vi "PH_TKTDS-30xx.set Channel GUI Element.vi"(0 "i ref in":refnum<vi>, 2 "GUI Element Name":string="N/A", 3 "Channel Config":T1={"Channel Name"="CH1", "Input Impedance"="MEG", "Max Input Frequency"="TWENTY", "Vertical Coupling"=1, "Channel Enabled"=TRUE, "Probe Attenuation"=1.0, "Vertical Range"=100.0, "Vertical Offset"=0.0, "Waveform Limits"={"Start"=1, "End"=10000}} {"Vertical Offset" format="%#_6p"; "Vertical Range" items=["1mV"=0.001, "2mV"=0.002, "5mV"=0.005, "10mV"=0.01, "20mV"=0.02, "50mV"=0.05, "100mV"=0.1, "200mV"=0.2, "500mV"=0.5, "1V"=1.0]; "Probe Attenuation" format="%#.2f"}, 5 "error in":errorcluster) -> (14 "i ref out":refnum<vi>, 19 "error out":errorcluster)   [LabVIEW 2014, in "PH_TKTDS-30xx.lvlib"]
doc: "If the reference is valid, the incoming data are set to the GUI."
uses:
  PH_TKTDS-30xx.lvlib
  PH_TKTDS-30xx.Channel Config.ctl
  PH_TKTDS-30xx.Waveform Limits.ctl
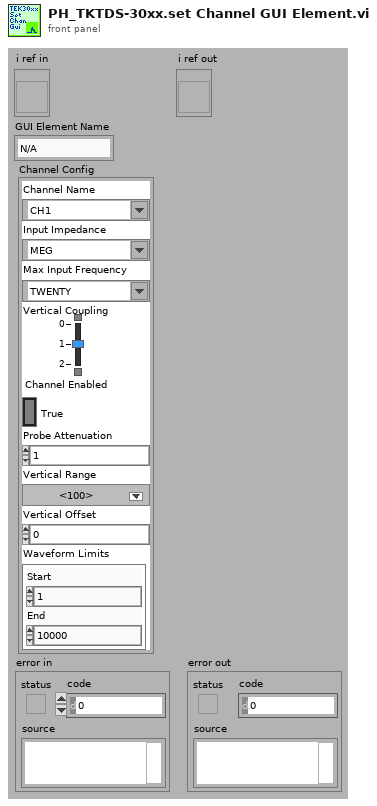
[diagram p1: front panel]
types:
  T1 = typedef "PH_TKTDS-30xx.lvlib/PH_TKTDS-30xx.Channel Config.ctl" = cluster{"Channel Name":string, "Input Impedance":string, "Max Input Frequency":string, "Vertical Coupling":i32, "Channel Enabled":bool, "Probe Attenuation":dbl, "Vertical Range":dbl, "Vertical Offset":dbl, "Waveform Limits":T2}
  T2 = typedef "PH_TKTDS-30xx.lvlib/PH_TKTDS-30xx.Waveform Limits.ctl" = cluster{"Start":i32, "End":i32}
  T3 = typedef "PH_TKTDS-30xx.lvlib/PH_TKTDS-30xx.i attribute.ctl" = cluster{"Default VISA Resource":string, "VISA Resource Name":refnum<visa-resource-name>, "Revision":cluster{"Instrument Driver":string, "Instrument Firmware":string}, "Selftest":cluster{"Result":u32, "Message":string}, "Channels":T1[], "Trigger Configuration":T4, "Acquisition Configuration":T5, "Fetched Waveforms":T6[], "GUI Refs":T7, "State":T8, "Error Message":string, "Allow Prdc Loop?":bool}
  T4 = typedef "PH_TKTDS-30xx.lvlib/PH_TKTDS-30xx.Trigger Config.ctl" = cluster{"Source":string, "Slope":i32, "Level [V]":dbl}
  T5 = typedef "PH_TKTDS-30xx.lvlib/PH_TKTDS-30xx.Acquisition Config.ctl" = cluster{"Time base":dbl, "Record Length":u16, "Start Time":dbl, "Type":i32, "Continuous":bool}
  T6 = typedef "PH_TKTDS-30xx.lvlib/PH_TKTDS-30xx.fetched Waveform.ctl" = cluster{"Source":string, "Actual Points":u32, "Initial X":dbl, "X Increment":dbl, "Waveform Array":dbl[]}
  T7 = typedef "PH_TKTDS-30xx.lvlib/PH_TKTDS-30xx.GUI Refs.ctl" = cluster{"Trigger":refnum<vi>, "Acquisition":refnum<vi>, "State":refnum<vi>, "Delete":refnum<vi>, "Channel to be positioned":refnum<vi>, "Postion":refnum<vi>, "Display Intensity":refnum<vi>, "VISA Resource":refnum<vi>, "Channels":refnum<vi>[], "Graphs":refnum<vi>[]}
  T8 = typedef "PH_StatusHandler.lvlib/PH_StatusHandler.Status.ctl" = i16
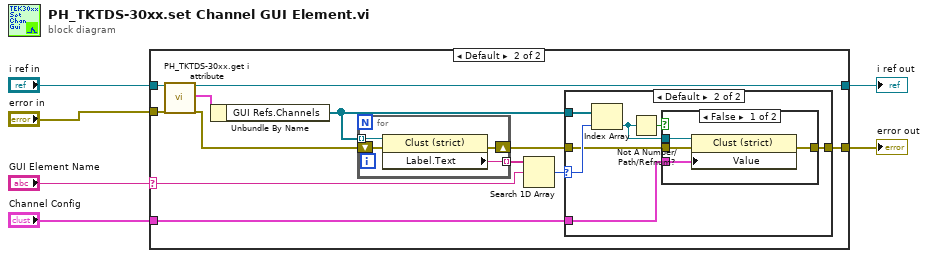
[diagram p0: block diagram]
diagram:
  n1 = case shown="Default" "GUI Element Name" {
    selector: "GUI Element Name" -> [_ w9]
    tunnel: "Channel Config" -> [_ w16]
    tunnel: [w7 w15] -> w5
    tunnel: "error in" -> [w7 w12]
    tunnel: "i ref in" -> [w8 w11]
    tunnel: [w8 w10] -> w2
    frame "", "N/A" {
    }
    frame Default {
      n2 = call "PH_TKTDS-30xx.get i attribute.vi"("i ref in"=w11, "error in (no error)"=w12) -> ("i ref out"=w10:refnum<vi>, "i attribute"=w14:T3, "error out"=w13:errorcluster)  [unwired: 15 in]
      n3 = Unbundle By Name(w14) -> ("GUI Refs.Channels"=w18:refnum<vi>[])
      n4 = for {
        tunnel: w18 -> [w37] mode=indexing
        tunnel: [w36] -> w20 mode=indexing
        shift-right: [w35] -> w17
        shift-left: w13 -> [w34]
        n5 = property class="Clust (strict)"(reference=w37, error in=w34) -> (error out=w35:errorcluster, "Label.Text"=w36:string)  [unwired: 1 out]
      }
      n6 = Search 1D Array(1D array=w20, element=w9) -> (index of element=w19:i32)  [unwired: 1 in]
      n7 = case shown="Default" w19 {
        selector: w19 -> [_ w27]
        tunnel: w18 -> [_ w28]
        tunnel: w17 -> [w21 w25]
        tunnel: w16 -> [_ w24]
        tunnel: [w21 w23] -> w15
        frame -1 {
        }
        frame Default {
          n8 = Index Array(array=w28, index=w27) -> (element=w26:refnum<vi>)
          n9 = Not A Number/Path/Refnum?(number/path/refnum=w26) -> (NaN/Path/Refnum?=w22:bool)
          n10 = case shown="False" w22 {
            tunnel: w25 -> [w32 w33]
            tunnel: [w31 w33] -> w23
            tunnel: w26 -> [w30 _]
            tunnel: w24 -> [w29 _]
            frame False {
              n11 = property class="Clust (strict)"(reference=w30, error in=w32, "Value"=w29) -> (error out=w31:errorcluster)  [unwired: 1 out]
            }
            frame True {
            }
          }
        }
      }
    }
  }
  "error out" <- w5
  "i ref out" <- w2
